vi "采集切换2.vi"(8 "error in (no error)":errorcluster, 11 "切换":bool) -> (0 "error out":errorcluster)   [LabVIEW 2020]
uses:
  Libraries/S7/S7.lvlib
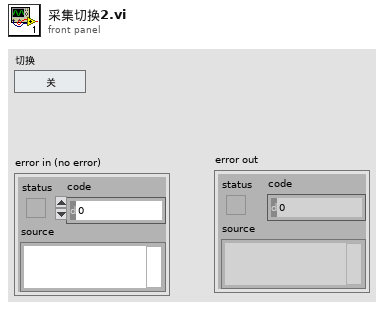
[diagram p1: front panel]
types:
  T1 = typedef "S7.lvlib/Read_Data (Reply Payload)--cluster.ctl" = cluster{"读取成功":bool, "数据":u32[], "Read_Data_error":errorcluster}
  T2 = cluster{"Boolean array[0]":bool, "Boolean array[1]":bool, "Boolean array[2]":bool, "Boolean array[3]":bool, "Boolean array[4]":bool, "Boolean array[5]":bool, "Boolean array[6]":bool, "Boolean array[7]":bool}
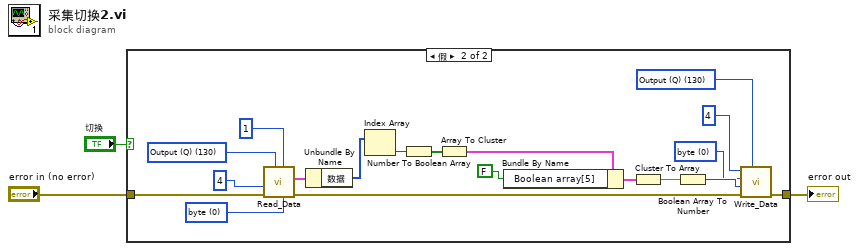
[diagram p0: block diagram]
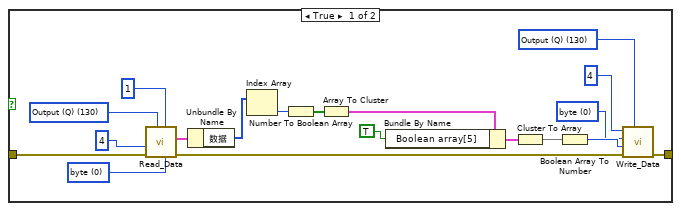
[diagram p2: hidden frame]
diagram:
  n1 = case shown="假" "切换" {
    tunnel: "error in (no error)" -> [w5 w24]
    tunnel: [w4 w23] -> w1
    frame True {
      w12 = u16 0 items=["byte", "word", "Dword"] ("数据类型")
      w10 = u8 130 items=["I/O (P)"=128, "Input (I)"=129, "Output (Q)"=130, "Bit Memory (M)"=131, "Data (DB)"=132, "Instance Data (DI)"=133, "Local Data (L)"=134, "Predecessor Local Data (VL)"=135] ("寄存器类型")
      w7 = u16 0 items=["byte", "word", "Dword"] ("数据类型")
      w8 = u8 130 items=["I/O (P)"=128, "Input (I)"=129, "Output (Q)"=130, "Bit Memory (M)"=131, "Data (DB)"=132, "Instance Data (DI)"=133, "Local Data (L)"=134, "Predecessor Local Data (VL)"=135] ("寄存器类型")
      n2 = call "Read_Data.vi"("数据类型"=w12, "读取长度"=u16 1, "寄存器类型"=w10, "error in (no error)"=w5, "起始地址"=u32 4) -> ("error out"=w22:errorcluster, "Reply Payload"=w15:T1)  [unwired: 4 in, 1 out]
      n3 = Unbundle By Name(w15) -> ("数据"=w14:u32[])
      n4 = Index Array(array=w14) -> (element=w17:u32)  [unwired: 1 in]
      n5 = Number To Boolean Array(number=w17) -> (Boolean array=w16:bool[])
      n6 = Array To Cluster(array=w16) -> (cluster=w18:T2)
      n7 = Bundle By Name(cluster=w18, "Boolean array[5]"=TRUE ("Boolean array[4]")) -> (w20:T2)
      n8 = Cluster To Array(cluster=w20) -> (array=w19:bool[])
      n9 = Boolean Array To Number(Boolean array=w19) -> (number=w21:u32)
      n10 = call "Write_Data.vi"("寄存器类型"=w8, "error in (no error)"=w22, "写入数据"=w21, "数据类型"=w7, "写入地址"=u32 4) -> ("error out"=w4:errorcluster)  [unwired: 4 in, 2 out]
    }
    frame False {
      w31 = u16 0 items=["byte", "word", "Dword"] ("数据类型")
      w29 = u8 130 items=["I/O (P)"=128, "Input (I)"=129, "Output (Q)"=130, "Bit Memory (M)"=131, "Data (DB)"=132, "Instance Data (DI)"=133, "Local Data (L)"=134, "Predecessor Local Data (VL)"=135] ("寄存器类型")
      w26 = u16 0 items=["byte", "word", "Dword"] ("数据类型")
      w27 = u8 130 items=["I/O (P)"=128, "Input (I)"=129, "Output (Q)"=130, "Bit Memory (M)"=131, "Data (DB)"=132, "Instance Data (DI)"=133, "Local Data (L)"=134, "Predecessor Local Data (VL)"=135] ("寄存器类型")
      n11 = call "Read_Data.vi"("数据类型"=w31, "读取长度"=u16 1, "寄存器类型"=w29, "error in (no error)"=w24, "起始地址"=u32 4) -> ("error out"=w41:errorcluster, "Reply Payload"=w34:T1)  [unwired: 4 in, 1 out]
      n12 = Unbundle By Name(w34) -> ("数据"=w33:u32[])
      n13 = Index Array(array=w33) -> (element=w36:u32)  [unwired: 1 in]
      n14 = Number To Boolean Array(number=w36) -> (Boolean array=w35:bool[])
      n15 = Array To Cluster(array=w35) -> (cluster=w37:T2)
      n16 = Bundle By Name(cluster=w37, "Boolean array[5]"=FALSE ("Boolean array[4]")) -> (w39:T2)
      n17 = Cluster To Array(cluster=w39) -> (array=w38:bool[])
      n18 = Boolean Array To Number(Boolean array=w38) -> (number=w40:u32)
      n19 = call "Write_Data.vi"("寄存器类型"=w27, "error in (no error)"=w41, "写入数据"=w40, "数据类型"=w26, "写入地址"=u32 4) -> ("error out"=w23:errorcluster)  [unwired: 4 in, 2 out]
    }
  }
  "error out" <- w1
